vi "CheckIOModule.vi"(6 "Timeout (ms)":u32=5000, 8 "error in (no error)":errorcluster, 11 "FPGA VI Reference In":T1) -> (0 "error out":errorcluster, 3 "FPGA VI Reference Out":T1)   [LabVIEW 2012]
uses:
  Common FPGA VIs/Basic_FPGA_Ref.ctl
  <vilib>/LabVIEW Targets/FPGA/FlexRIO/CustomFPGAMethods/79XXR_Method_IOModuleStatusImpl.vi
  <vilib>/rvi/interface/nirviMethod/nirviMethod.xnode
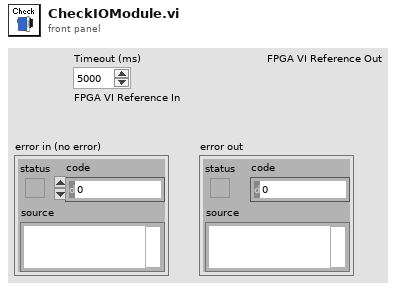
[diagram p1: front panel]
types:
  T1 = typedef "Basic_FPGA_Ref.ctl" = refnum<k20>
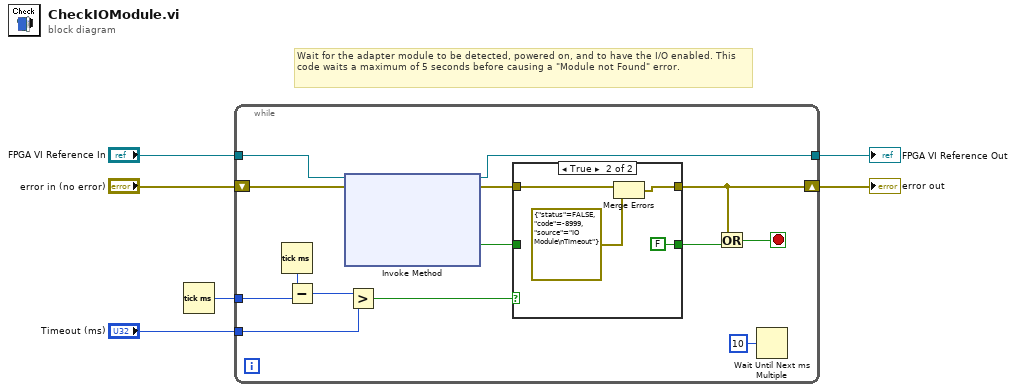
[diagram p0: block diagram]
diagram:
  # "Wait for the adapter module to be detected, powered on, and to have the I/O enabled. This code waits a maximum of 5 seconds before causing a \"Module not Found\" error."
  n1 = Tick Count (ms)() -> (millisecond timer value=w4:u32)
  n2 = while {
    tunnel: "FPGA VI Reference In" -> [w20]
    tunnel: w4 -> [w17]
    shift-right: [w11] -> w5
    shift-left: "error in (no error)" -> [w19]
    tunnel: [w9] -> w1
    tunnel: "Timeout (ms)" -> [w7]
    stop <- w10 stop-if-true
    n3 = Tick Count (ms)() -> (millisecond timer value=w18:u32)
    n4 = Subtract(x=w18, y=w17) -> (x-y=w16:u32)
    n5 = xnode "Invoke Method"("FPGA VI Reference In"=w20, "error in"=w19) -> ("FPGA VI Reference Out"=w9:T1, "error out"=w14:errorcluster, "IO Enabled?"=w13:bool)  [unwired: 3 out]
    n6 = Greater?(x=w16, y=w7) -> (0:w15:bool)
    n7 = case shown="True" w15 {
      tunnel: w14 -> [w22 w25]
      tunnel: [w22 w24] -> w11
      tunnel: w13 -> [w21 _]
      tunnel: [w21 FALSE ("IO Enabled?")] -> w12
      frame False {
      }
      frame True {
        n8 = Merge Errors(w25, errorcluster {"status"=FALSE, "code"=-8999, "source"="IO Module\nTimeout"} ("error out")) -> (w24:errorcluster)
      }
    }
    n9 = Or(x=w11, y=w12) -> (x .or. y?=w10:bool)
    n10 = Wait Until Next ms Multiple(millisecond multiple=u32 10) -> ()  [unwired: 1 out]
  }
  "error out" <- w5
  "FPGA VI Reference Out" <- w1
